vi "Untitled 3 (SubVI).vi"(11 "Output bit stream":i8[](array[numeric])) -> (3 "Array":string[](array[string]))   [LabVIEW 2018]
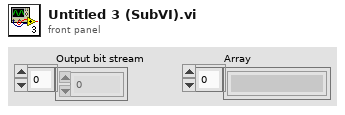
[diagram p1: front panel]
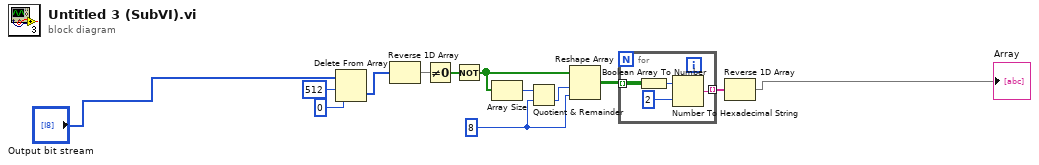
[diagram p0: block diagram]
diagram:
  w2 = 8 ("dimension size")
  n1 = Delete From Array(array="Output bit stream", length=512, index=0) -> (deleted portion=w9:i8[])  [unwired: 1 out]
  n2 = Reverse 1D Array(array=w9) -> (reversed array=w6:i8[])
  n3 = Not Equal To 0?(x=w6) -> (x != 0?=w12:bool[])
  n4 = Not(x=w12) -> (.not. x?=w13:bool[])
  n5 = Array Size(array=w13) -> (size(s)=w3:i32)
  n6 = Quotient & Remainder(x=w3, y=w2) -> (floor(x/y)=w4:i32)  [unwired: 1 out]
  n7 = Reshape Array(w13, w4, w2) -> (w1:bool[][])
  n8 = for {
    tunnel: w1 -> [w15] mode=indexing
    tunnel: [w16] -> w5 mode=indexing
    n9 = Boolean Array To Number(Boolean array=w15) -> (number=w17:u32)
    n10 = Number To Hexadecimal String(1:i8 2, 2:w17) -> (0:w16:string)
  }
  n11 = Reverse 1D Array(array=w5) -> (reversed array=→"Array":string[])
